vi "3D-CalMaxValue.vi"(10 "ROI Array":T1[](array[typedef]) {"Rotation" format="%.2f"; "Left" scale=0.0..1024.0; "Right" scale=0.0..1024.0}, 11 "Image Pixels (U8)A":dbl[][](array[numeric])=[[1.0, 2.0, 3.0, 4.0, 5.0, 6.0], [2.0, 3.0, 4.0, 5.0, 6.0, 7.0], [3.0, 4.0, 5.0, 6.0, 7.0, 8.0], [4.0, 5.0, 6.0, 7.0, 8.0, 9.0], [5.0, 6.0, 7.0, 8.0, 9.0, 10.0]]) -> (0 "XY index":i32[][](array[numeric]), 1 "XY index":cluster{"X":dbl, "Y":dbl}[](array[cluster]), 3 "Max Value":string[][](array[string]))   [LabVIEW 2015]
panel:
  out "Image Pixels (U8)A 2":dbl[][](array[numeric])
  out "最大值":u8
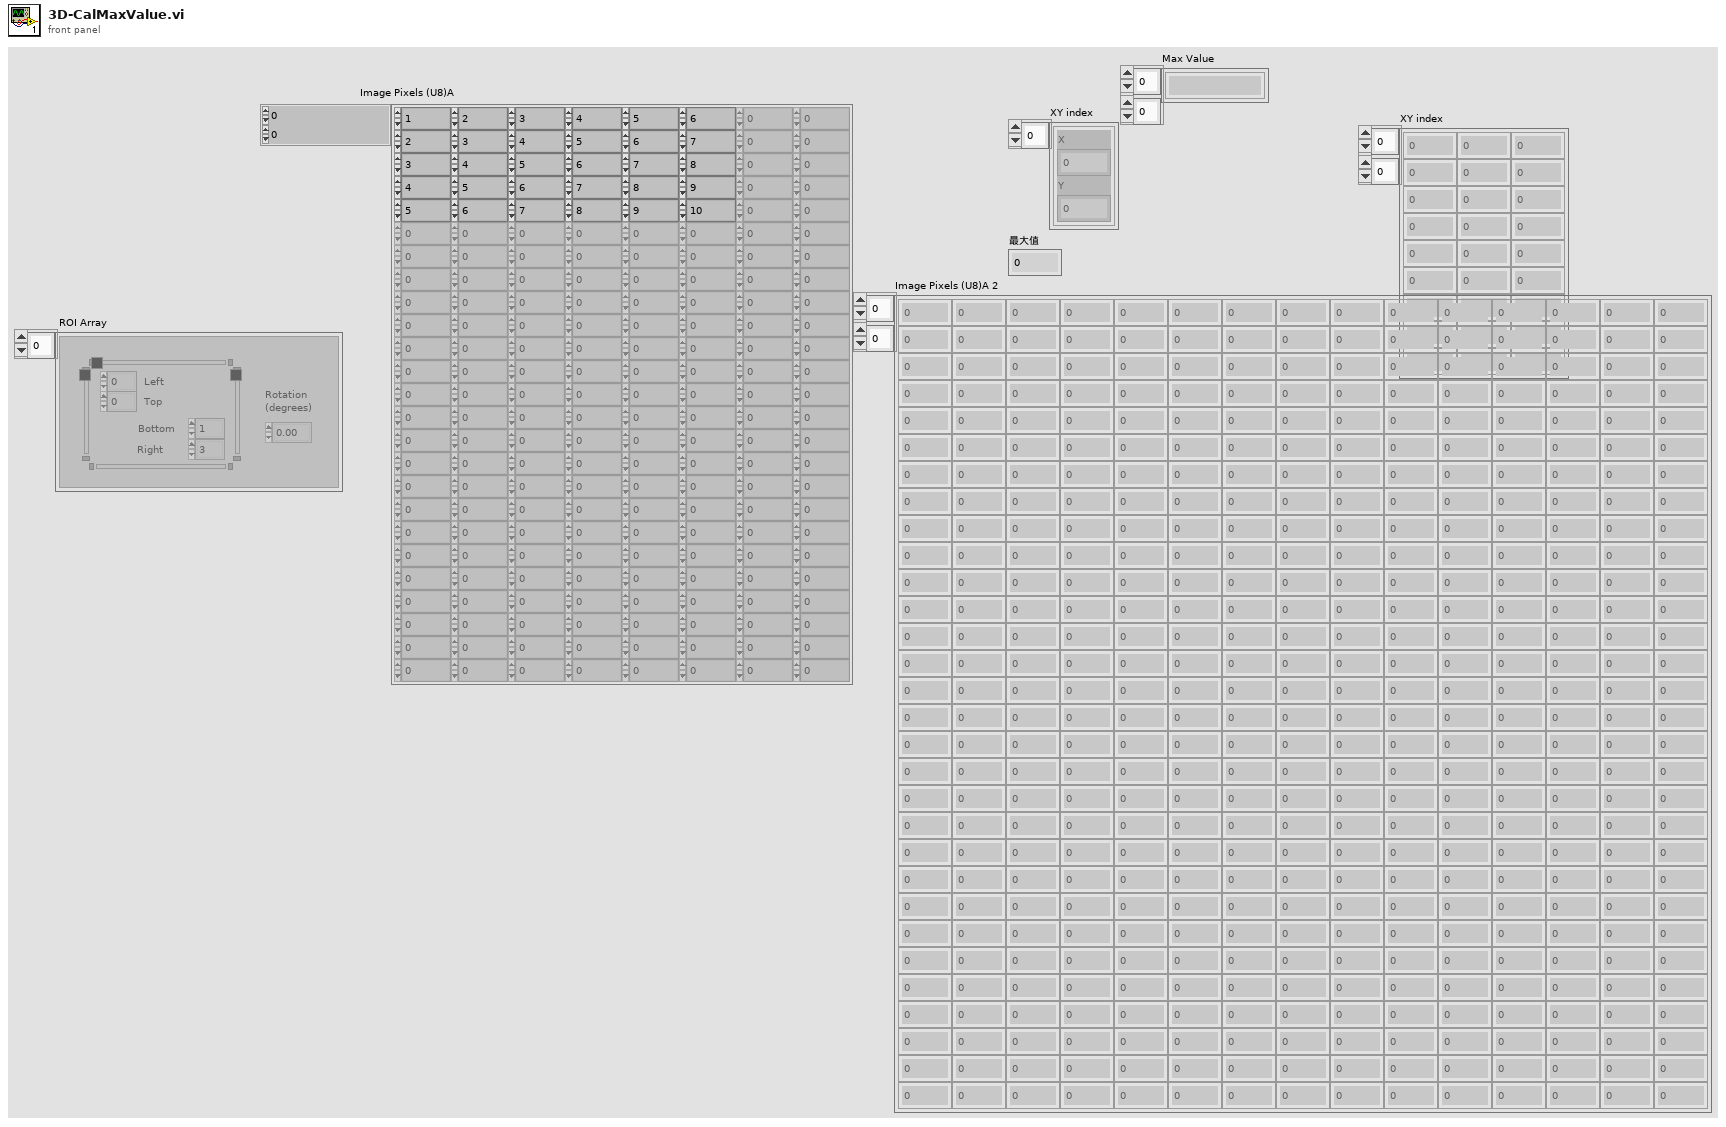
[diagram p1: front panel]
types:
  T1 = typedef "IMAQ Rectangle" = cluster{"Left":i32, "Top":i32, "Right":i32, "Bottom":i32, "Rotation":dbl}
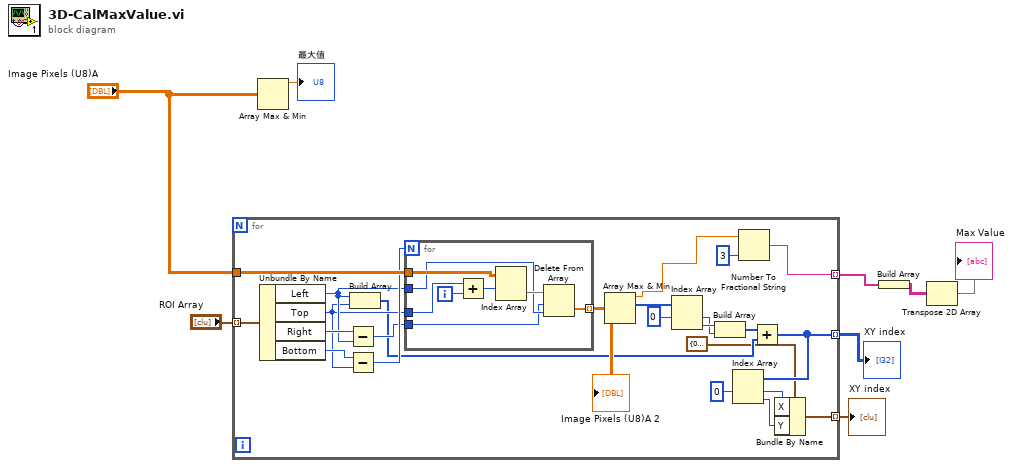
[diagram p0: block diagram]
diagram:
  n1 = for {
    tunnel: "ROI Array" -> [w32] mode=indexing
    tunnel: "Image Pixels (U8)A" -> [w30]
    tunnel: [w17] -> w7 mode=indexing
    tunnel: [w15] -> w6 mode=indexing
    tunnel: [w12] -> w5 mode=indexing
    n2 = Unbundle By Name(w32) -> ("Left"=w25:i32, "Top"=w24:i32, "Right"=w31:i32, "Bottom"=w28:i32)
    n3 = Subtract(x=w31, y=w25) -> (x-y=w27:i32)
    n4 = Subtract(x=w28, y=w24) -> (x-y=w29:i32)
    n5 = Build Array(w25, w24) -> (w23:i32[])
    n6 = for {
      N: w29 -> [_]
      tunnel: w30 -> [w40]
      tunnel: w24 -> [w39]
      tunnel: w25 -> [w35]
      tunnel: w27 -> [w34]
      tunnel: [w33] -> w26 mode=indexing
      i -> [w38]
      n7 = Add(x=w39, y=w38) -> (x+y=w37:i32)
      n8 = Index Array(array=w40, index (row)=w37) -> (element=w36:dbl[])  [unwired: 1 in]
      n9 = Delete From Array(array=w36, length=w34, index=w35) -> (deleted portion=w33:dbl[])  [unwired: 1 out]
    }
    "Image Pixels (U8)A 2" <- w26
    n10 = Array Max & Min(array=w26) -> (max value=w14:dbl, max index (indices)=w22:i32[])  [unwired: 2 out]
    n11 = Index Array(array=w22, index #1=0 ("索引")) -> (element #1=w19:i32, element #2=w20:i32)  [unwired: 1 in]
    n12 = Build Array(w20, w19) -> (w18:i32[])
    n13 = Number To Fractional String(number=w14, precision (6)=i16 3 ("精度(6)")) -> (F-format string=w12:string)  [unwired: 2 in]
    n14 = Add(x=w18, y=w23) -> (x+y=w17:i32[])
    n15 = Index Array(array=w17, index #1=0 ("索引")) -> (element #1=w9:i32, element #2=w10:i32)  [unwired: 1 in]
    n16 = Bundle By Name(cluster=cluster{"X":dbl, "Y":dbl} {"X"=0.0, "Y"=0.0} ("输入簇"), "X"=w9, "Y"=w10) -> (w15:cluster{"X":dbl, "Y":dbl})
  }
  "XY index" <- w7
  "XY index" <- w6
  n17 = Array Max & Min(array="Image Pixels (U8)A") -> (max value=→"最大值":dbl)  [unwired: 3 out]
  n18 = Build Array(w5) -> (w4:string[][])
  n19 = Transpose 2D Array(2D array=w4) -> (transposed array=→"Max Value":string[][])
